vi "Livebild.vi"(8 "Fehler in":errorcluster, 11 "Cluster in":T2={"Initialisierung"={"Online?"=FALSE, "Grundpfad"=path "", "Kamera Oben"="", "IP-Adresse Flüssiglinse"="", "Flüssiglinse"=refnum, "Kamera Unten"="", "IP-Adresse SPS"="", "SPS-Verbindung"={"TCP Connection Ref"=refnum, "IP address"="", "timeout ms"=5000, "Connected?"=FALSE, "PLC Type"=enum."S7 1200", "Rack S7 400"=0, "Slot S7 400"=0, "PDU Size"=0, "connection semaphore"=refnum}, "IP-Adresse Lichtgitter"="", "Lichtgitter"=refnum, "Skalierungsfaktor"=0.0, "Bilder Oben"=[], "Bild Unten"=refnum, "Bild Ausschnitt Unten"=refnum}, "Einstellungen"={"Gesamtablauf gestartet"=FALSE, "i. O. Bilder speichern"=FALSE, "Bildspeicherung Offline"=FALSE, "Ausgewähltes Offline-Datum"="", "Ausgewähltes Offline-Teil"="", "Speicherpfad Bilder"=path ""}, "Artikeldaten"={"Artikelnummer"="", "Fertigungsauftrag"="", "Muster ISO"=refnum, "Belichtungszeit Referenzmarken"=0.0, "Fokus Referenzmarken"=0.0, "Belichtungszeit ISO"=0.0, "Fokus ISO"=0.0, "Belichtungszeit Unten"=0.0, "Kontaktanzahl"=0, "Aktueller Kontakt"=0, "Kontaktposition"={"x"=0.0, "y"=0.0}, "Winkel ISO"=0.0, "ISO-Muster nicht vorhanden"=FALSE}, "Werte Kamera Oben"={"Koordinatensystem"={"Punkt x-Achse"={"X"=0.0, "Y"=0.0}, "Ursprung"={"X"=0.0, "Y"=0.0}, "Punkt y-Achse"={"X"=0.0, "Y"=0.0}}, "Position Kontakt"={"x"=0.0, "y"=0.0}, "Winkel Kontakt"=0.0}, "Werte Kamera Unten"={"Prüfung Unten n. i. O."=FALSE}, "Werte Lichtgitter"={"Messwerte Referenzmarken"=[], "Mittelpunkt Referenzmarken"={"x"=0.0, "y"=0.0}, "Messwerte Kontakt"=[], "Offset"={"x"=0.0, "y"=0.0}}, "Rückmeldungen"={"Koordinaten ermittelt"=FALSE, "Vermessung Lichtgitter fertig"=FALSE, "Nachkontrolle Kamera Unten fertig"=FALSE}, "Fehler"={"Referenzen nicht gefunden"=FALSE, "Kontakt nicht gefunden"=FALSE, "Referenzen nicht in Lichtgitter"=FALSE, "Kontakt zu groß"=FALSE, "Kontakt zu klein"=FALSE}, "Statistik"={"Statistiken"=[]}, "Timer"={"Timer Start Position"=0, "Timer Start Lichtgitter"=0, "Timer Start Kamera Unten"=0}}) -> (0 "Fehler out":errorcluster, 3 "Cluster out":T2={"Initialisierung"={"Online?"=FALSE, "Grundpfad"=path "", "Kamera Oben"="", "IP-Adresse Flüssiglinse"="", "Flüssiglinse"=refnum, "Kamera Unten"="", "IP-Adresse SPS"="", "SPS-Verbindung"={"TCP Connection Ref"=refnum, "IP address"="", "timeout ms"=5000, "Connected?"=FALSE, "PLC Type"=enum."S7 1200", "Rack S7 400"=0, "Slot S7 400"=0, "PDU Size"=0, "connection semaphore"=refnum}, "IP-Adresse Lichtgitter"="", "Lichtgitter"=refnum, "Skalierungsfaktor"=0.0, "Bilder Oben"=[], "Bild Unten"=refnum, "Bild Ausschnitt Unten"=refnum}, "Einstellungen"={"Gesamtablauf gestartet"=FALSE, "i. O. Bilder speichern"=FALSE, "Bildspeicherung Offline"=FALSE, "Ausgewähltes Offline-Datum"="", "Ausgewähltes Offline-Teil"="", "Speicherpfad Bilder"=path ""}, "Artikeldaten"={"Artikelnummer"="", "Fertigungsauftrag"="", "Muster ISO"=refnum, "Belichtungszeit Referenzmarken"=0.0, "Fokus Referenzmarken"=0.0, "Belichtungszeit ISO"=0.0, "Fokus ISO"=0.0, "Belichtungszeit Unten"=0.0, "Kontaktanzahl"=0, "Aktueller Kontakt"=0, "Kontaktposition"={"x"=0.0, "y"=0.0}, "Winkel ISO"=0.0, "ISO-Muster nicht vorhanden"=FALSE}, "Werte Kamera Oben"={"Koordinatensystem"={"Punkt x-Achse"={"X"=0.0, "Y"=0.0}, "Ursprung"={"X"=0.0, "Y"=0.0}, "Punkt y-Achse"={"X"=0.0, "Y"=0.0}}, "Position Kontakt"={"x"=0.0, "y"=0.0}, "Winkel Kontakt"=0.0}, "Werte Kamera Unten"={"Prüfung Unten n. i. O."=FALSE}, "Werte Lichtgitter"={"Messwerte Referenzmarken"=[], "Mittelpunkt Referenzmarken"={"x"=0.0, "y"=0.0}, "Messwerte Kontakt"=[], "Offset"={"x"=0.0, "y"=0.0}}, "Rückmeldungen"={"Koordinaten ermittelt"=FALSE, "Vermessung Lichtgitter fertig"=FALSE, "Nachkontrolle Kamera Unten fertig"=FALSE}, "Fehler"={"Referenzen nicht gefunden"=FALSE, "Kontakt nicht gefunden"=FALSE, "Referenzen nicht in Lichtgitter"=FALSE, "Kontakt zu groß"=FALSE, "Kontakt zu klein"=FALSE}, "Statistik"={"Statistiken"=[]}, "Timer"={"Timer Start Position"=0, "Timer Start Lichtgitter"=0, "Timer Start Kamera Unten"=0}})   [LabVIEW 2024]
doc: "Zeigt das Livebild der Kameras an. Außerdem könnne die Belichtungszeiten und bei der oberen Kamera zusätzlich die Fokusebene verändert werden."
uses:
  Cluster.ctl
  Kontaktmontagemodul.exe/1abvi3w/vi.lib/userDefined/High Color/IMAQdx.ctl
  Kontaktmontagemodul.exe/1abvi3w/vi.lib/DATA AHEAD/SP7/typedefs/S7 Connection.ctl
  Kontaktmontagemodul.exe/1abvi3w/vi.lib/DATA AHEAD/SP7/typedefs/PLC Type.ctl
  Kontaktmontagemodul.exe/1abvi3w/vi.lib/vision/Image Controls.llb/IMAQ Image.ctl
  Koordinatensystem.ctl
  Statistik.ctl
  Kontaktmontagemodul.exe/1abvi3w/vi.lib/vision/driver/NI_Vision_Acquisition_Software.lvlib
  <resource>/objmgr/imaqdx.rc
  Kontaktmontagemodul.exe/1abvi3w/vi.lib/DATA AHEAD/SP7/SP7.lvlib
panel:
  in  "Lichtgitterposition anzeigen":bool
  in  "Zoom zurücksetzen":bool
  out "Fehler Live":errorcluster
  in  "Fokusebene":sgl(slide) min=-2 max=3.5 step=0.01 scale=-2.0..3.5
  in  "Kamera Oben/Unten":bool
  in  "Speicherpfad öffnen":bool
  in  "Bild speichern":bool
  in  "Belichtungszeit":u32(slide) max=100000 scale=0.0..100000.0
  out "Livebild":T1(plugin-control)
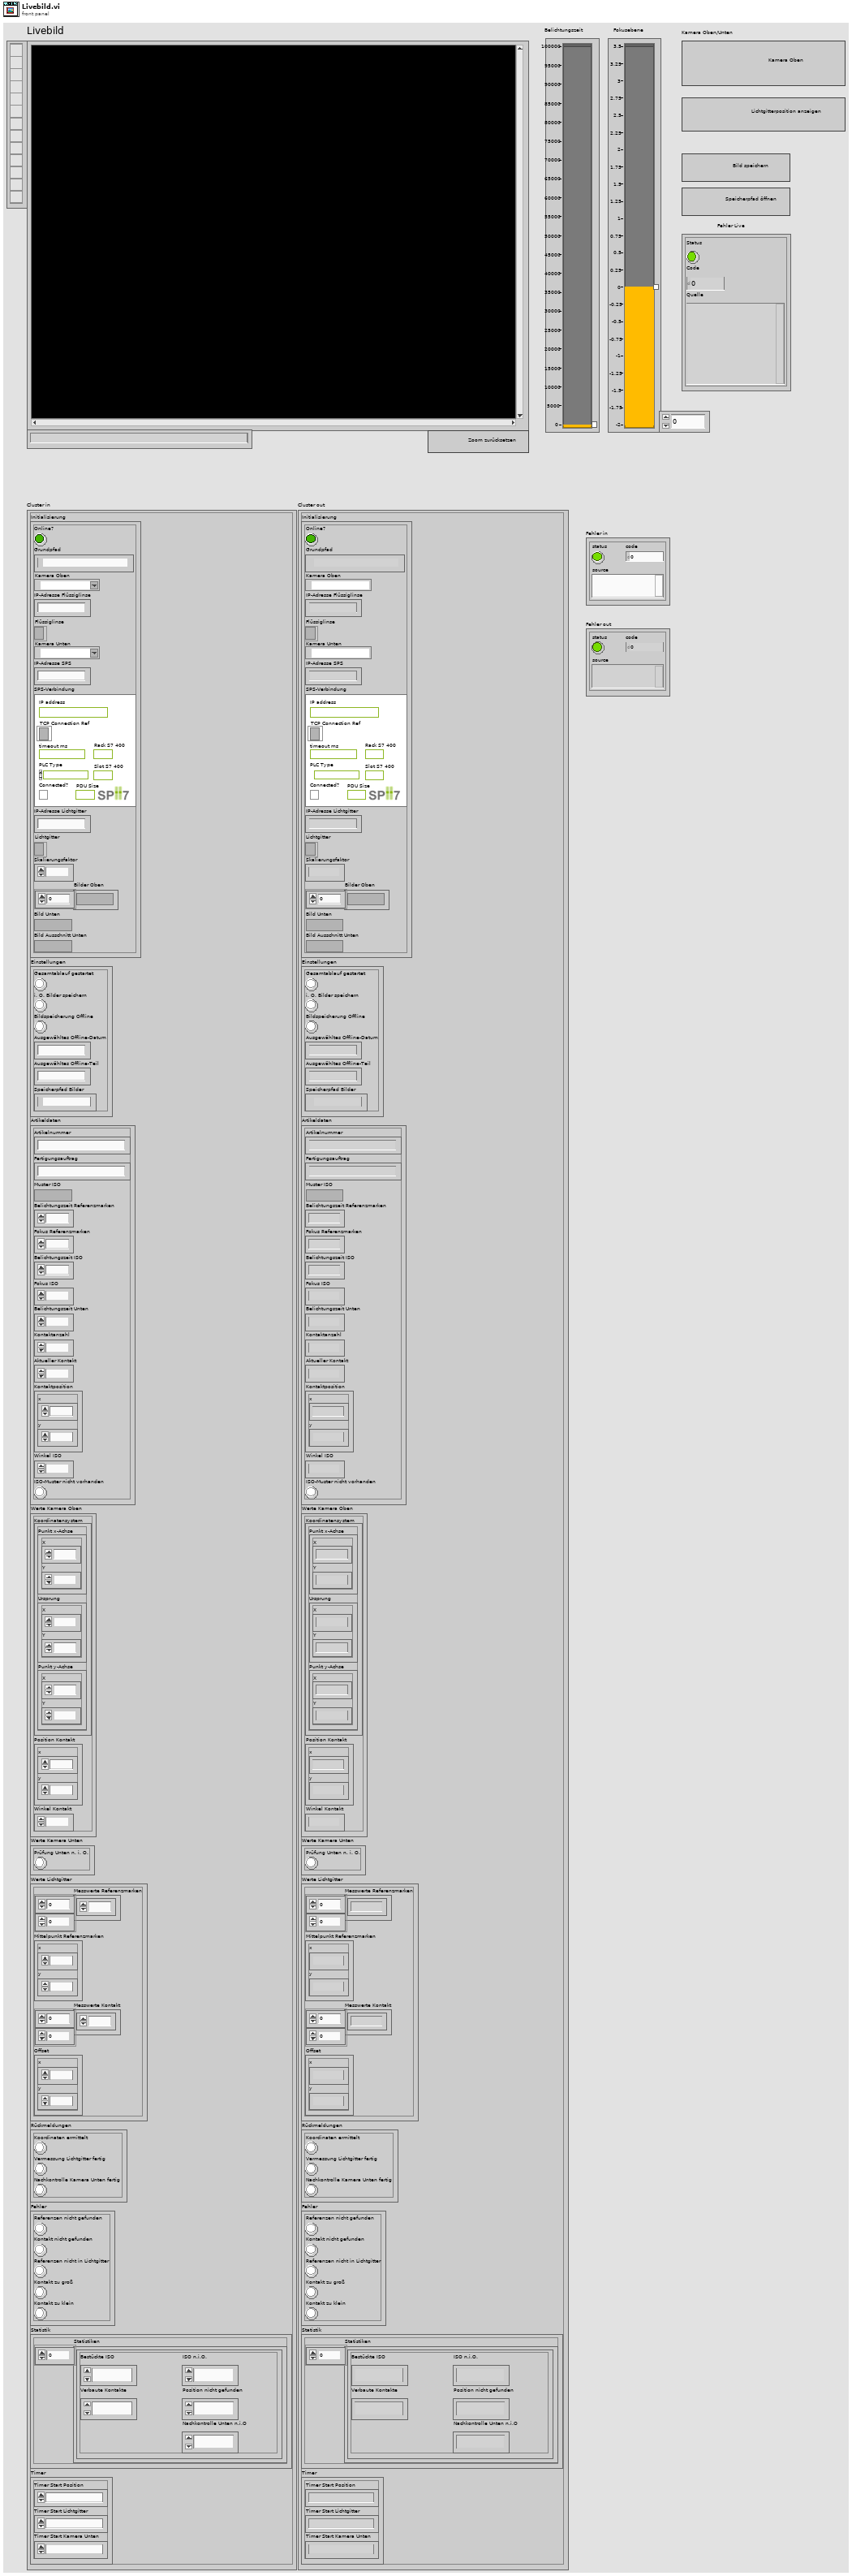
[diagram p1: front panel]
types:
  T1 = typedef "IMAQ Image.ctl" = refnum<image>
  T2 = typedef "Cluster.ctl" = cluster{"Initialisierung":cluster{"Online?":bool, "Grundpfad":path, "Kamera Oben":T3, "IP-Adresse Flüssiglinse":string, "Flüssiglinse":refnum<k5>, "Kamera Unten":T3, "IP-Adresse SPS":string, "SPS-Verbindung":T4, "IP-Adresse Lichtgitter":string, "Lichtgitter":refnum<k5>, "Skalierungsfaktor":dbl, "Bilder Oben":T1[], "Bild Unten":T1, "Bild Ausschnitt Unten":T1}, "Einstellungen":cluster{"Gesamtablauf gestartet":bool, "i. O. Bilder speichern":bool, "Bildspeicherung Offline":bool, "Ausgewähltes Offline-Datum":string, "Ausgewähltes Offline-Teil":string, "Speicherpfad Bilder":path}, "Artikeldaten":cluster{"Artikelnummer":string, "Fertigungsauftrag":string, "Muster ISO":T1, "Belichtungszeit Referenzmarken":dbl, "Fokus Referenzmarken":dbl, "Belichtungszeit ISO":dbl, "Fokus ISO":dbl, "Belichtungszeit Unten":dbl, "Kontaktanzahl":u32, "Aktueller Kontakt":i16, "Kontaktposition":cluster{"x":sgl, "y":sgl}, "Winkel ISO":sgl, "ISO-Muster nicht vorhanden":bool}, "Werte Kamera Oben":cluster{"Koordinatensystem":T7, "Position Kontakt":cluster{"x":dbl, "y":dbl}, "Winkel Kontakt":dbl}, "Werte Kamera Unten":cluster{"Prüfung Unten n. i. O.":bool}, "Werte Lichtgitter":cluster{"Messwerte Referenzmarken":dbl[][], "Mittelpunkt Referenzmarken":cluster{"x":dbl, "y":dbl}, "Messwerte Kontakt":dbl[][], "Offset":cluster{"x":dbl, "y":dbl}}, "Rückmeldungen":cluster{"Koordinaten ermittelt":bool, "Vermessung Lichtgitter fertig":bool, "Nachkontrolle Kamera Unten fertig":bool}, "Fehler":cluster{"Referenzen nicht gefunden":bool, "Kontakt nicht gefunden":bool, "Referenzen nicht in Lichtgitter":bool, "Kontakt zu groß":bool, "Kontakt zu klein":bool}, "Statistik":cluster{"Statistiken":T8[]}, "Timer":cluster{"Timer Start Position":u32, "Timer Start Lichtgitter":u32, "Timer Start Kamera Unten":u32}}
  T3 = typedef "IMAQdx.ctl" = refnum<k21>
  T4 = typedef "SP7.lvlib/S7 Connection.ctl" = cluster{"TCP Connection Ref":refnum<k5>, "IP address":string, "timeout ms":i32, "Connected?":bool, "PLC Type":T5, "Rack S7 400":u8, "Slot S7 400":u8, "PDU Size":u16, "connection semaphore":T6}
  T5 = typedef "SP7.lvlib/PLC Type.ctl" = enum16{"S7 200", "S7 300/400", "S7 1200", "S7 1500", "LOGO!8"}
  T6 = typedef "Semaphore RefNum" = refnum<k1>
  T7 = typedef "Koordinatensystem.ctl" = cluster{"Punkt x-Achse":cluster{"X":sgl, "Y":sgl}, "Ursprung":cluster{"X":sgl, "Y":sgl}, "Punkt y-Achse":cluster{"X":sgl, "Y":sgl}}
  T8 = typedef "Statistik.ctl" = cluster{"Bestückte ISO":u32, "Verbaute Kontakte":u32, "ISO n.i.O.":u32, "Nachkontrolle Unten n.i.O":u32, "Position nicht gefunden":u32}
  T9 = enum8{"Enabled", "Disabled", "Disabled and Grayed Out"}
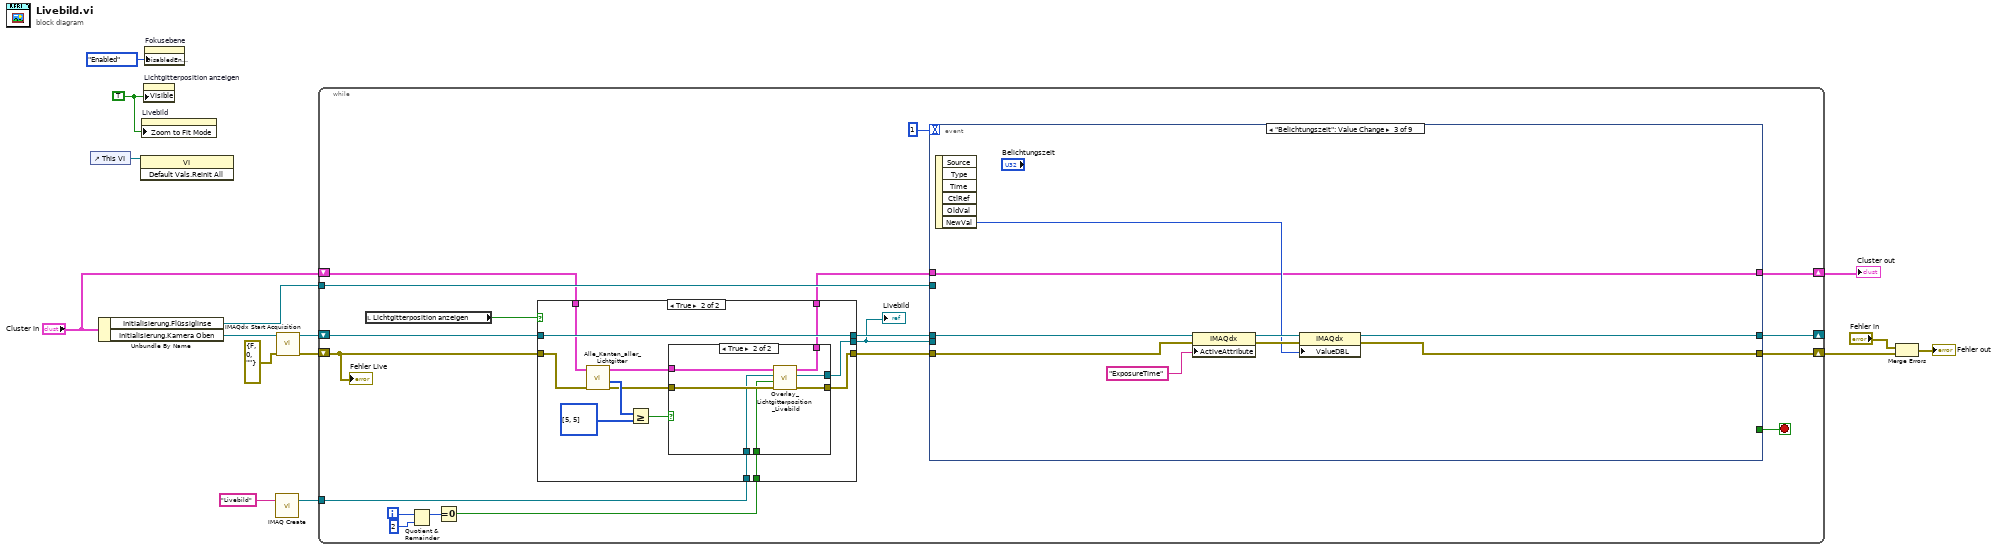
[diagram p0: block diagram]
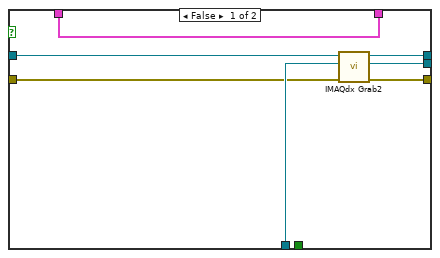
[diagram p2: hidden frame]
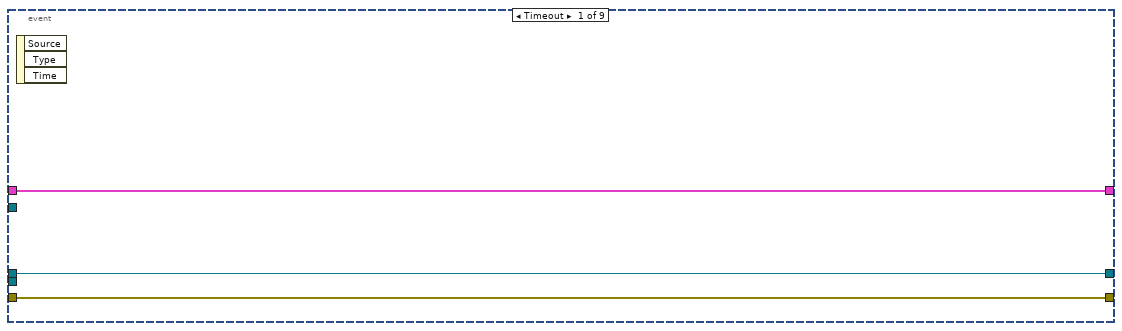
[diagram p4: hidden frame]
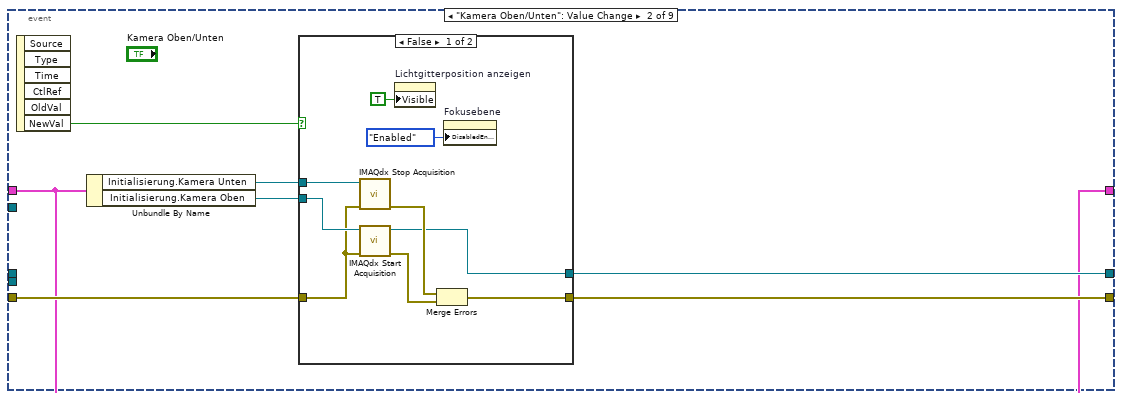
[diagram p5: hidden frame]
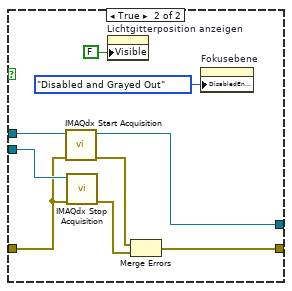
[diagram p6: hidden frame]
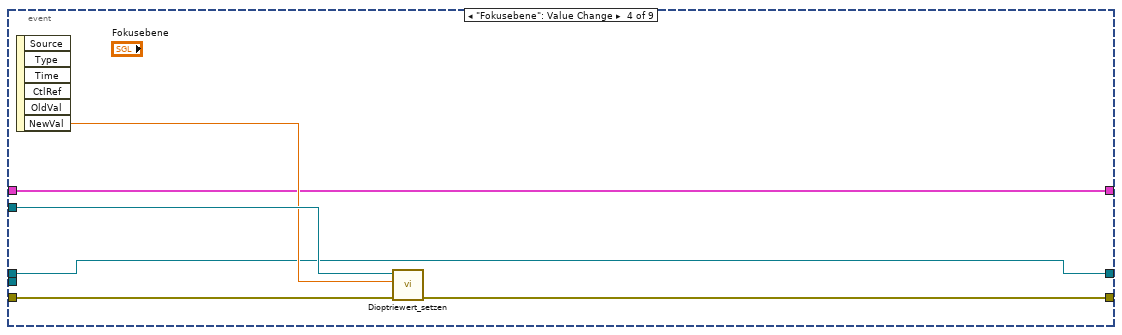
[diagram p7: hidden frame]
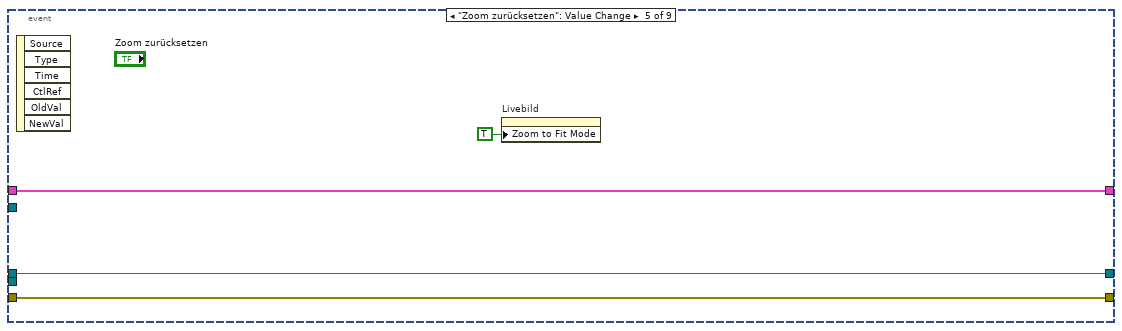
[diagram p8: hidden frame]
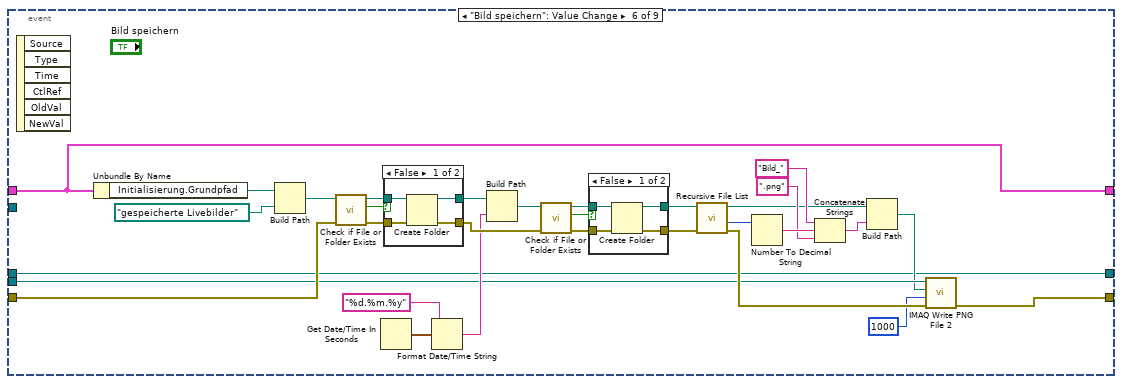
[diagram p9: hidden frame]
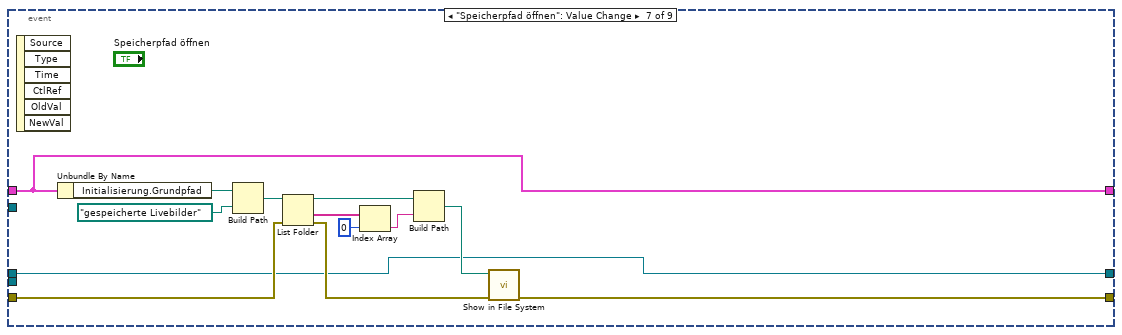
[diagram p12: hidden frame]
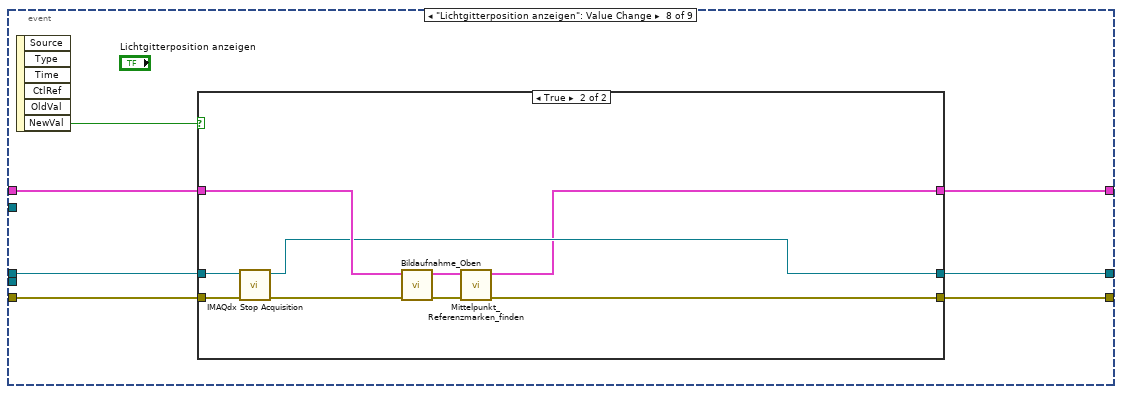
[diagram p13: hidden frame]
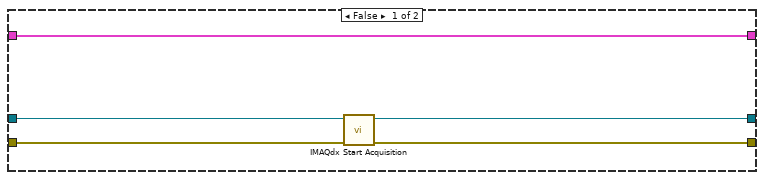
[diagram p14: hidden frame]
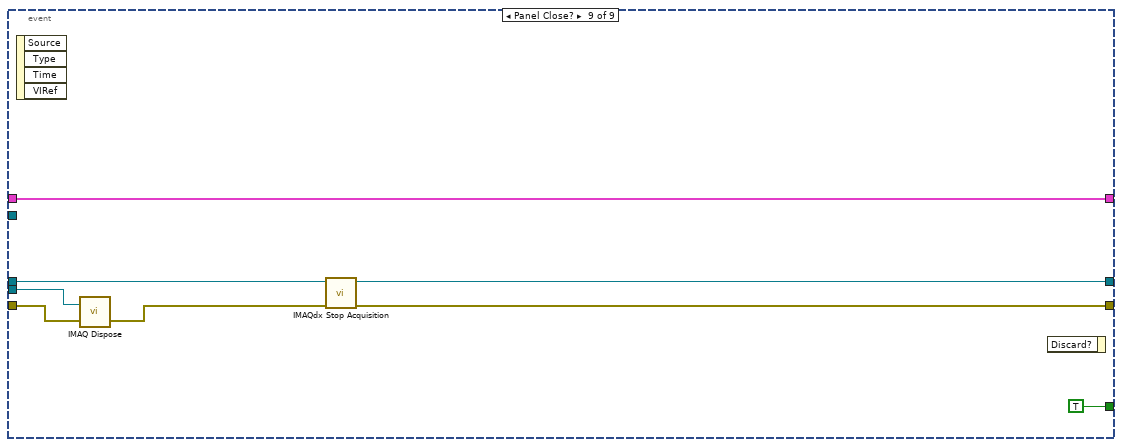
[diagram p15: hidden frame]
diagram:
  w2 = TRUE ("Visible")
  n1 = control-ref of="This VI"() -> (w15:refnum<vi>)
  n2 = Unbundle By Name("Cluster in") -> ("Initialisierung.Flüssiglinse"=w5:refnum<k5>, "Initialisierung.Kamera Oben"=w13:T3)
  n3 = invoke class="VI" method="Default Vals.Reinit All"(reference=w15) -> ()  [unwired: 2 in, 3 out]
  n4 = property on="Livebild" class="ImageControl"("Zoom to Fit Mode"=w2) -> ()  [unwired: 2 in, 2 out]
  n5 = property on="Lichtgitterposition anzeigen" class="Bool (strict)"("Visible"=w2) -> ()  [unwired: 2 in, 2 out]
  n6 = property on="Fokusebene" class="Slide (strict)"("DisabledEnum"=T9."Enabled" ("Disabled")) -> ()  [unwired: 2 in, 2 out]
  n7 = call "IMAQ Create"("Image Name"="Livebild") -> ("New Image"=w9:T1)  [unwired: 4 in, 1 out]
  n8 = call "IMAQdx Start Acquisition.vi"("error in"=errorcluster {"status"=FALSE, "code"=0, "source"=""} ("Fehler"), "Session In"=w13) -> ("error out"=w11:errorcluster, "Session Out"=w12:T3)  [unwired: 8 in]
  n9 = while {
    shift-right: [w31] -> _
    shift-left: w12 -> [w33]
    shift-right: [w28] -> w7
    shift-left: w11 -> [w26]
    tunnel: w9 -> [w32]
    tunnel: w5 -> [w27]
    shift-right: [w23] -> w1
    shift-left: "Cluster in" -> [w21]
    i -> [w19]
    stop <- w30 stop-if-true
    n10 = local read "Lichtgitterposition anzeigen"() -> (w22:bool)
    n11 = Quotient & Remainder(x=w19, y=2) -> (x-y*floor(x/y)=w17:i32)  [unwired: 1 out]
    n12 = Equal To 0?(x=w17) -> (x = 0?=w16:bool)
    n13 = case shown="True" w22 {
      tunnel: w33 -> [w41 w54]
      tunnel: w32 -> [w40 w51]
      tunnel: [w39 w54] -> w29
      tunnel: w26 -> [w38 w47]
      tunnel: [w37 w50] -> w25
      tunnel: [w36 w52] -> w24
      tunnel: w21 -> [w35 w48]
      tunnel: [w35 w43] -> w20
      tunnel: w16 -> [_ w42]
      frame False {
        n14 = call "IMAQdx Grab2.vi"("error in"=w38, "Image In"=w40, "Session In"=w41) -> ("error out"=w36:errorcluster, "Image Out"=w37:T1, "Session Out"=w39:T3)  [unwired: 5 in, 1 out]
      }
      frame True {
        n15 = call "Alle_Kanten_aller_Lichtgitter.vi"("Fehler in"=w47, "Cluster in"=w48) -> ("Fehler out"=w45:errorcluster, "Anzahl Kanten"=w46:i32[], "Cluster out"=w44:T2)  [unwired: 6 in, 1 out]
        n16 = Greater Or Equal?(x=w46, y=i32[] [5, 5]) -> (x >= y?=w49:bool)
        n17 = case shown="True" w49 {
          tunnel: [w56 w60] -> w52
          tunnel: w51 -> [w57 w62]
          tunnel: [w57 w61] -> w50
          tunnel: w45 -> [w56 w64]
          tunnel: w44 -> [w55 w63]
          tunnel: [w55 w59] -> w43
          tunnel: w42 -> [_ w58]
          frame False {
          }
          frame True {
            n18 = call "Overlay_Lichtgitterposition _Livebild.vi"("error in"=w64, "gerade?"=w58, "Image in"=w62, "Cluster in"=w63) -> ("error out"=w60:errorcluster, "Image out"=w61:T1, "Cluster out"=w59:T2)  [unwired: 5 in]
          }
        }
      }
    }
    "Livebild" <- w25
    n19 = event shown="[2] \"Belichtungszeit\": Value Change" {
      selector: _ -> [_ _ _ _ _ _ _ _ _]
      dyn-events: _ -> [_ _ _ _ _ _ _ _ _]
      timeout: 1 -> [_ _ _ _ _ _ _ _ _]
      tunnel: w20 -> [w65 w68 w93 w102 w108 w112 w155 w174 w189]
      tunnel: [w67 w69 w94 w103 w110 w113 w156 w171 w194] -> w31
      tunnel: [_ _ _ _ _ _ _ _ TRUE] -> w30
      tunnel: w29 -> [w67 _ w98 w103 w110 w113 w156 w173 w195]
      tunnel: w24 -> [w66 w71 w97 w106 w109 w137 w160 w172 w191]
      tunnel: [w66 w70 w95 w105 w109 w114 w157 w169 w193] -> w28
      tunnel: w25 -> [_ _ _ _ _ w119 _ _ w192]
      tunnel: w27 -> [_ _ _ w107 _ _ _ _ _]
      tunnel: [w65 w68 w93 w102 w108 w112 w155 w170 w189] -> w23
      event Timeout {
        n20 = event-data() -> ()  [unwired: 1 in, 3 out]
      }
      event "Kamera Oben/Unten": Value Change {
        n21 = event-data() -> ("NewVal"=w74:bool)  [unwired: 1 in, 5 out]
        n22 = Unbundle By Name(w68) -> ("Initialisierung.Kamera Unten"=w72:T3, "Initialisierung.Kamera Oben"=w73:T3)
        n23 = case shown="False" w74 {
          tunnel: w73 -> [w83 w92]
          tunnel: w72 -> [w82 w91]
          tunnel: w71 -> [w81 w90]
          tunnel: [w79 w87] -> w70
          tunnel: [w77 w86] -> w69
          frame False {
            n24 = call "IMAQdx Stop Acquisition.vi"("error in"=w81, "Session In"=w82) -> ("error out"=w78:errorcluster)  [unwired: 8 in, 1 out]
            n25 = call "IMAQdx Start Acquisition.vi"("error in"=w81, "Session In"=w83) -> ("error out"=w80:errorcluster, "Session Out"=w77:T3)  [unwired: 8 in]
            n26 = property on="Lichtgitterposition anzeigen" class="Bool (strict)"("Visible"=TRUE) -> ()  [unwired: 2 in, 2 out]
            n27 = Merge Errors(w78, w80) -> (w79:errorcluster)
            n28 = property on="Fokusebene" class="Slide (strict)"("DisabledEnum"=T9."Enabled" ("Disabled")) -> ()  [unwired: 2 in, 2 out]
          }
          frame True {
            n29 = call "IMAQdx Start Acquisition.vi"("error in"=w90, "Session In"=w91) -> ("error out"=w89:errorcluster, "Session Out"=w86:T3)  [unwired: 8 in]
            n30 = call "IMAQdx Stop Acquisition.vi"("error in"=w90, "Session In"=w92) -> ("error out"=w88:errorcluster)  [unwired: 8 in, 1 out]
            n31 = property on="Lichtgitterposition anzeigen" class="Bool (strict)"("Visible"=FALSE) -> ()  [unwired: 2 in, 2 out]
            n32 = Merge Errors(w89, w88) -> (w87:errorcluster)
            n33 = property on="Fokusebene" class="Slide (strict)"("DisabledEnum"=T9."Disabled and Grayed Out" ("Disabled")) -> ()  [unwired: 2 in, 2 out]
          }
        }
      }
      event "Belichtungszeit": Value Change {
        n34 = event-data() -> ("NewVal"=w96:u32)  [unwired: 1 in, 5 out]
        n35 = property class="IMAQdx"(reference=w98, error in=w97, "ActiveAttribute"="ExposureTime") -> (reference out=w100:T3, error out=w101:errorcluster)
        n36 = property class="IMAQdx"(reference=w100, error in=w101, "ValueDBL"=w96) -> (reference out=w94:T3, error out=w95:errorcluster)
      }
      event "Fokusebene": Value Change {
        n37 = event-data() -> ("NewVal"=w104:sgl)  [unwired: 1 in, 5 out]
        n38 = call "Dioptriewert_setzen.vi"("Fehler in"=w106, "Dioptrie-Wert"=w104, "Flüssiglinse in"=w107) -> ("Fehler out"=w105:errorcluster)  [unwired: 7 in, 1 out]
      }
      event "Zoom zurücksetzen": Value Change {
        n39 = event-data() -> ()  [unwired: 1 in, 6 out]
        n40 = property on="Livebild" class="ImageControl"("Zoom to Fit Mode"=TRUE) -> ()  [unwired: 2 in, 2 out]
      }
      event "Bild speichern": Value Change {
        n41 = event-data() -> ()  [unwired: 1 in, 6 out]
        n42 = Unbundle By Name(w112) -> ("Initialisierung.Grundpfad"=w142:path)
        n43 = Build Path(base path=w142, name or relative path=path "gespeicherte Livebilder") -> (appended path=w140:path)
        n44 = call "Check if File or Folder Exists.vi"("error in (no error)"=w137, "path"=w140) -> ("error out"=w136:errorcluster, "file or folder exists?"=w139:bool, "dup path"=w138:path)  [unwired: 7 in]
        n45 = Get Date/Time In Seconds() -> (seconds since 1Jan1904=w135:timestamp)
        n46 = case shown="False" w139 {
          tunnel: w138 -> [w151 w154]
          tunnel: w136 -> [w152 w153]
          tunnel: [w150 w154] -> w130
          tunnel: [w149 w153] -> w128
          frame False {
            n47 = Create Folder(path (use dialog)=w151, error in=w152) -> (created path=w150:path, error out=w149:errorcluster)  [unwired: 1 in, 1 out]
          }
          frame True {
          }
        }
        n48 = Format Date/Time String(time format string (%c)="%d.%m.%y", seconds (now)=w135) -> (date/time string=w127:string)  [unwired: 1 in]
        n49 = Build Path(base path=w130, name or relative path=w127) -> (appended path=w129:path)
        n50 = call "Check if File or Folder Exists.vi"("error in (no error)"=w128, "path"=w129) -> ("error out"=w133:errorcluster, "file or folder exists?"=w131:bool, "dup path"=w132:path)  [unwired: 7 in]
        n51 = case shown="False" w131 {
          tunnel: w132 -> [w145 w148]
          tunnel: w133 -> [w146 w147]
          tunnel: [w144 w148] -> w126
          tunnel: [w143 w147] -> w125
          frame False {
            n52 = Create Folder(path (use dialog)=w145, error in=w146) -> (created path=w144:path, error out=w143:errorcluster)  [unwired: 1 in, 1 out]
          }
          frame True {
          }
        }
        n53 = call "Recursive File List.vi"("error in (no error)"=w125, "Folder Path"=w126) -> ("error out"=w120:errorcluster, "Number of Files"=w124:i32, "dup Folder Path"=w118:path)  [unwired: 5 in, 2 out]
        n54 = Number To Decimal String(number=w124) -> (decimal integer string=w122:string)  [unwired: 1 in]
        n55 = Concatenate Strings("Bild_" ("time format string (%c)"), w122, ".png" ("string")) -> (w117:string)
        n56 = Build Path(base path=w118, name or relative path=w117) -> (appended path=w116:path)
        n57 = call "IMAQ Write PNG File 2"("error in (no error)"=w120, "Image Quality"=u32 1000, "File Path"=w116, "Image"=w119) -> ("error out"=w114:errorcluster)  [unwired: 6 in, 1 out]
      }
      event "Speicherpfad öffnen": Value Change {
        n58 = event-data() -> ()  [unwired: 1 in, 6 out]
        n59 = Unbundle By Name(w155) -> ("Initialisierung.Grundpfad"=w166:path)
        n60 = Build Path(base path=w166, name or relative path=path "gespeicherte Livebilder") -> (appended path=w165:path)
        n61 = List Folder(path=w165, error in=w160) -> (path out=w162:path, folder names=w164:string[], error out=w158:errorcluster)  [unwired: 2 in, 1 out]
        n62 = Index Array(array=w164, index=0) -> (element=w161:string)
        n63 = Build Path(base path=w162, name or relative path=w161) -> (appended path=w159:path)
        n64 = call "Show in File System.vi"("error in (no error)"=w158, "file or directory path"=w159) -> ("error out"=w157:errorcluster)  [unwired: 9 in]
      }
      event "Lichtgitterposition anzeigen": Value Change {
        n65 = event-data() -> ("NewVal"=w168:bool)  [unwired: 1 in, 5 out]
        n66 = case shown="True" w168 {
          tunnel: w174 -> [w179 w187]
          tunnel: w173 -> [w178 w186]
          tunnel: w172 -> [w177 w185]
          tunnel: [w176 w183] -> w171
          tunnel: [w179 w180] -> w170
          tunnel: [w175 w182] -> w169
          frame False {
            n67 = call "IMAQdx Start Acquisition.vi"("error in"=w177, "Session In"=w178) -> ("error out"=w175:errorcluster, "Session Out"=w176:T3)  [unwired: 8 in]
          }
          frame True {
            n68 = call "IMAQdx Stop Acquisition.vi"("error in"=w185, "Session In"=w186) -> ("error out"=w184:errorcluster, "Session Out"=w183:T3)  [unwired: 8 in]
            n69 = call "Bildaufnahme_Oben.vi"("Fehler in"=w184, "Cluster in"=w187) -> ("Fehler out"=w188:errorcluster, "Cluster out"=w181:T2)  [unwired: 8 in]
            n70 = call "Mittelpunkt_Referenzmarken_finden.vi"("Fehler in"=w188, "Cluster in"=w181) -> ("Fehler out"=w182:errorcluster, "Cluster out"=w180:T2)  [unwired: 7 in, 1 out]
          }
        }
      }
      event Panel Close? {
        n71 = event-data() -> ()  [unwired: 1 in, 4 out]
        n72 = call "IMAQ Dispose"("Image"=w192, "error in (no error)"=w191) -> ("error out"=w190:errorcluster)  [unwired: 4 in]
        n73 = call "IMAQdx Stop Acquisition.vi"("error in"=w190, "Session In"=w195) -> ("error out"=w193:errorcluster, "Session Out"=w194:T3)  [unwired: 8 in]
        n74 = event-data() -> ()  [unwired: 2 in, 1 out]
      }
    }
    "Fehler Live" <- w26
  }
  "Cluster out" <- w1
  n75 = Merge Errors("Fehler in", w7) -> (→"Fehler out":errorcluster)
